vi "Reset Laser.vi"(8 "error in (no error)":errorcluster, 11 "VISA Refnum in":refnum<visa-resource-name>) -> (0 "error out":errorcluster, 3 "VISA Refnum out":refnum<visa-resource-name>)   [LabVIEW 2016]
doc: "Resets the Hokuyo URG-04LX and empties the VISA communication buffers."
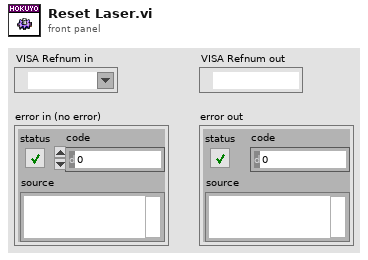
[diagram p1: front panel]
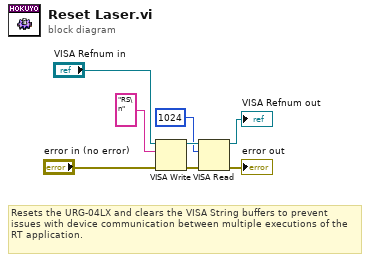
[diagram p0: block diagram]
diagram:
  # "Resets the URG-04LX and clears the VISA String buffers to prevent \nissues with device communication between multiple executions of the RT application."
  n1 = VISA Write(VISA resource name="VISA Refnum in", write buffer="RS\n", error in (no error)="error in (no error)") -> (VISA resource name out=w7:refnum<visa-resource-name>, error out=w3:errorcluster)  [unwired: 1 out]
  n2 = VISA Read(VISA resource name=w7, byte count=u32 1024, error in (no error)=w3) -> (VISA resource name out=→"VISA Refnum out":refnum<visa-resource-name>, error out=→"error out":errorcluster)  [unwired: 2 out]
